vi "Process.vi"(8 "error in (no error)":errorcluster, 10 "DAQ Class.lvclass":refnum<class "DAQ Class.lvclass">, 11 "Intensity Processing in":refnum<class "Intensity Processing.lvclass">) -> (0 "error out":errorcluster, 3 "Intensity Processing out":refnum<class "Intensity Processing.lvclass">)   [LabVIEW 2014, in "Intensity Processing.lvclass"]
uses:
  Intensity Processing.lvclass
  Classes/DAQ/DAQ Class.lvclass
  Classes/DAQ Control Functional Global States.ctl
  <vilib>/Analysis/4window.llb/Hanning Window (DBL).vi
  <vilib>/Analysis/2dsp.llb/Real FFT.vi
  <vilib>/Analysis/4window.llb/AllCosWindow (DBL).vi
  Classes/Processing.lvclass
  <vilib>/Analysis/NI_AALPro.lvlib
panel:
  out "Log?":bool=TRUE
  out "Intensity Graph":dbl[][](graph)
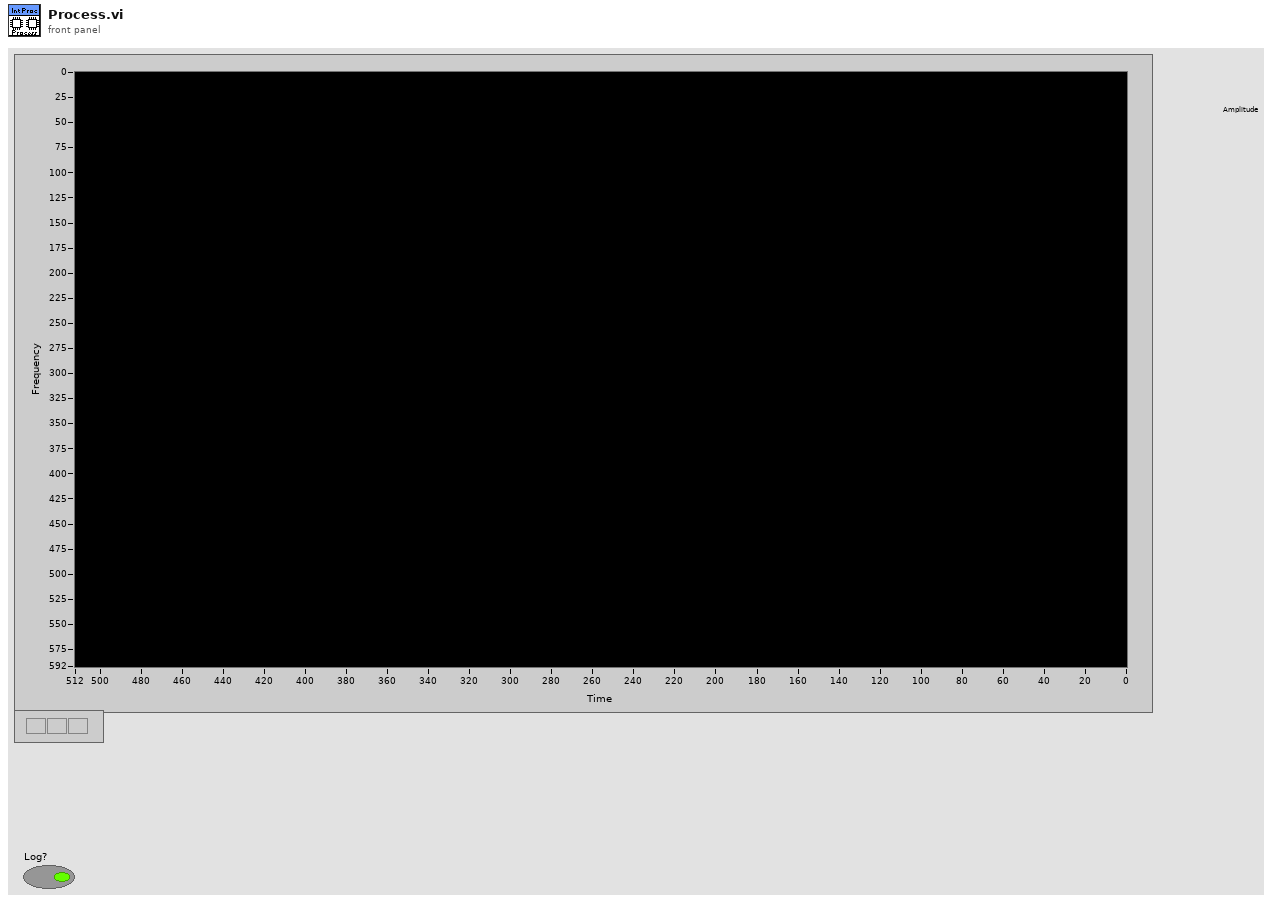
[diagram p1: front panel]
types:
  T1 = typedef "DAQ Class.lvclass/DAQ Parameters.ctl" = cluster{"Points Per A-Scan":u32, "A-Scans Per B-Scan":u32, "Number of B-Scans":u32, "A-Scans Per Transfer":u32, "Trigger Voltage":sgl, "Trigger Source":T2, "Trigger Slope":T3, "Channel":T4, "Clock":T5, "Bits per Sample":dbl, "Range":dbl}
  T2 = typedef "DAQ Class.lvclass/Trigger Source.ctl" = enum16{"External", "Channel A", "Channel B"}
  T3 = typedef "DAQ Class.lvclass/Trigger Slope.ctl" = enum16{"Rising", "Falling"}
  T4 = typedef "OCT DAQ Channel Data Type.ctl" = enum16{"Channel 1", "Channel 2", "Channel 1 and 2"}
  T5 = typedef "DAQ Class.lvclass/Clock Control.ctl" = enum16{"Internal Clock", "External Clock"}
  T6 = enum16{"open", "replace", "create", "open or create", "replace or create", "replace or create with confirmation"}
  T7 = typedef "DAQ Control Functional Global States.ctl" = enum16{"Status", "Set Processing Finished", "Reset", "Clear", "Set DAQ Finished"}
  T8 = typedef "LVCursorListTypeDef.ctl" = cluster{"Name":string, "Color":u32, "Style":u8, "Point Style":u8, "Name Visible":bool, "Allow Drag":bool, "Cursor Mode":u32, "Plot":i32, "Index":i32, "Position":cluster{"X":dbl, "Y":dbl}, "X Scale":u32, "Y Scale":u32, "Watch Plots":i32[], "Watch All Plots":bool, "Plot Area":i32, "Label Offset":cluster{"X":dbl, "Y":dbl}}[]
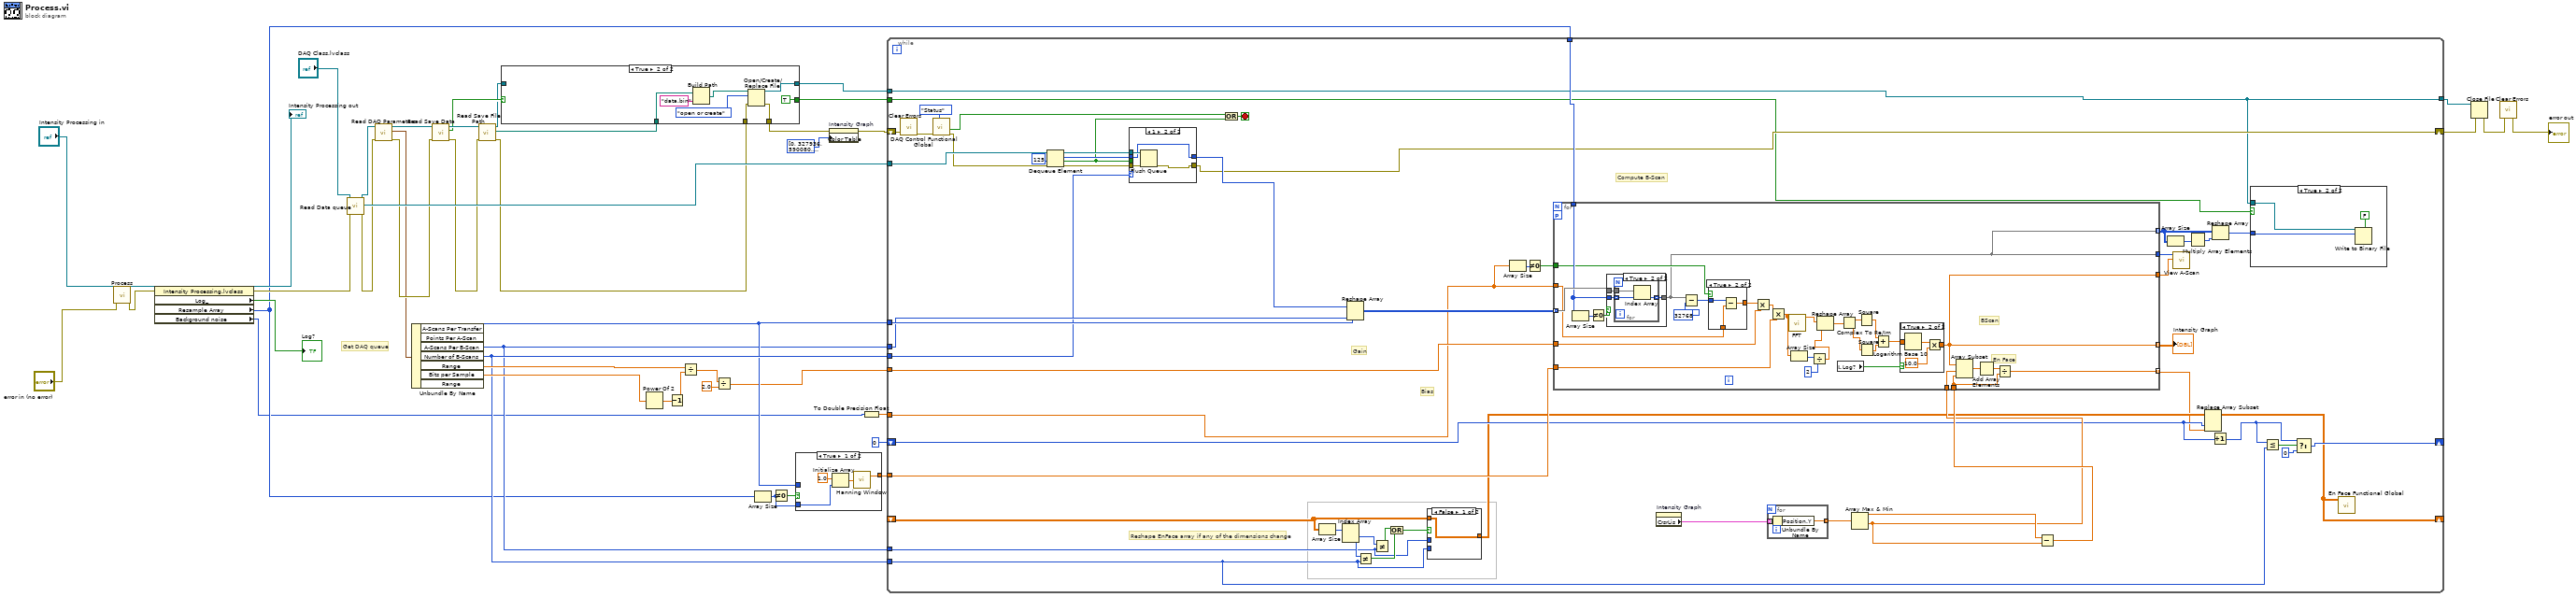
[diagram p0: block diagram]
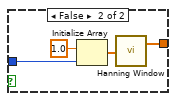
[diagram p2: hidden frame]
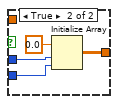
[diagram p9: hidden frame]
diagram:
  # "Get DAQ queue"
  n1 = call-parent "Process.vi"("error in (no error)"="error in (no error)", "Processing in"="Intensity Processing in") -> ("error out"=w24:errorcluster, "Processing out"=w26:refnum<class "Intensity Processing.lvclass">)  [unwired: 8 in]
  n2 = property class="Intensity Processing.lvclass"(reference=w26, error in=w24) -> (reference out=→"Intensity Processing out":refnum<class "Intensity Processing.lvclass">, error out=w23:errorcluster, "Log_"=→"Log?":bool, "Resample Array"=w7:u32[], "Background noise"=w1:u32[])
  n3 = call-dynamic "Read Data queue.vi"("error in (no error)"=w23, "DAQ Class in"="DAQ Class.lvclass") -> ("error out"=w44:errorcluster, "Data queue"=w45:refnum<queue>, "DAQ Class out"=w43:refnum<class "DAQ Class.lvclass">)  [unwired: 7 in]
  n4 = call-dynamic "Read DAQ Parameters.vi"("error in (no error)"=w44, "DAQ Class in"=w43) -> ("error out"=w19:errorcluster, "DAQ Parameters"=w9:T1, "DAQ Class out"=w21:refnum<class "DAQ Class.lvclass">)  [unwired: 7 in]
  n5 = Unbundle By Name(w9) -> ("Points Per A-Scan"=w14:u32, "A-Scans Per B-Scan"=w13:u32, "Number of B-Scans"=w15:u32, "Range"=w40:dbl, "Bits per Sample"=w41:dbl)  [unwired: 2 out]
  n6 = call-dynamic "Read Save Data.vi"("error in (no error)"=w19, "DAQ Class in"=w21) -> ("error out"=w20:errorcluster, "Save Data"=w17:bool, "DAQ Class out"=w18:refnum<class "DAQ Class.lvclass">)  [unwired: 7 in]
  n7 = call-dynamic "Read Save File Path.vi"("error in (no error)"=w20, "DAQ Class in"=w18) -> ("error out"=w33:errorcluster, "Save File Path"=w16:path, "DAQ Class out"=w5:refnum<class "DAQ Class.lvclass">)  [unwired: 7 in]
  n8 = case shown="True" w17 {
    selector: w17 -> [w47 _]
    tunnel: w33 -> [w48 w56]
    tunnel: [w48 w55] -> w11
    tunnel: [_ w54] -> w37
    tunnel: [w47 TRUE] -> w36
    tunnel: w16 -> [_ w52]
    tunnel: w5 -> [_ _]
    frame False {
    }
    frame True {
      n9 = Build Path(base path=w52, name or relative path="data.bin") -> (appended path=w51:path)
      n10 = Open/Create/Replace File(file path (use dialog)=w51, error in=w56, operation (0:open)=T6."open or create") -> (refnum out=w54:refnum<file>, error out=w55:errorcluster)  [unwired: 3 in, 1 out]
    }
  }
  n11 = Power Of 2(x=w41) -> (2^x=w42:dbl)
  n12 = Decrement(x=w42) -> (x-1=w39:dbl)
  n13 = Divide(x=w40, y=w39) -> (x/y=w4:dbl)
  n14 = Divide(x=w4, y=2.0) -> (x/y=w3:dbl)
  n15 = Array Size(array=w7) -> (size(s)=w6:i32)
  n16 = Not Equal To 0?(x=w6) -> (x != 0?=w8:bool)
  n17 = case shown="True" w8 {
    tunnel: [w58 w62] -> w31
    tunnel: w14 -> [_ w61]
    tunnel: w6 -> [w57 _]
    frame True {
      n18 = Initialize Array(1.0 ("element"), w57) -> (w60:dbl[])
      n19 = call-poly <vilib>:"Hanning Window.vi"("X"=w60) -> ("Windowed X"=w58:dbl[])  [unwired: 1 out]
    }
    frame False {
      n20 = Initialize Array(1.0 ("element"), w61) -> (w64:dbl[])
      n21 = call-poly <vilib>:"Hanning Window.vi"("X"=w64) -> ("Windowed X"=w62:dbl[])  [unwired: 1 out]
    }
  }
  n22 = property on="Intensity Graph" class="IntGraph (strict)"(error in=w11, "Color Table"=u32[] [0, 327936, 590080, 852224, 983296, 1114624, 1180160, 1311232, 1442304, 1573632, 1704704, 1770240, 1901312, 1966848, 2098176, 2163712, 2294784, 2491392, 2557184, 2688256, 2753792, 2884864, 2950656, 3081728, 3147264, 3344129, 3475457, 3540993, 3672321, 3738113, 3869185, 3934977, 4066305, 4197633, 4328961, 4394497, 4460289, 4591617, 4657409, 4788481, 4854273, 4985601, 5116929, 5248257, 5314049, 5379841, 5511169, 5576961, 5708033, 5773825, 5905153, 6036482, 6167810, 6233346, 6299138, 6430466, 6496258, 6562050, 6693634, 6759426, 6890754, 7022082, 7087874, 7153666, 7284994, 7350786, 7482114, 7547906, 7613698, 7745026, 7876354, 8007682, 8073474, 8139522, 8205314, 8336642, 8467970, 8533763, 8599555, 8665347, 8731139, 8862467, 8993795, 9059587, 9125380, 9191428, 9257220, 9388548, 9454340, 9520132, 9585924, 9717253, 9848837, 9914629, 9980165, 10045957, 10177541, 10243334, 10309126, 10375174, 10440966, 10572294, 10703623, 10769416, 10835208, 10901256, 10967049, 11033097, 11033609, 11099401, 11165450, 11231242, 11231754, 11297547, 11363339, 11429131, 11495180, 11495692, 11561740, 11693069, 11758861, 11759373, 11825165, 11891214, 11957006, 12022799, 12023311, 12089103, 12220944, 12286736, 12286736, 12352529, 12418577, 12484370, 12550162, 12615954, 12681747, 12747796, 12813588, 12813845, 12879894, 12945686, 13077015, 13142808, 13143064, 13208856, 13274905, 13340697, 13340953, 13472282, 13538075, 13604379, 13670172, 13735964, 13801757, 13867550, 13933343, 13999392, 13999648, 14065441, 14131234, 14197027, 14197541, 14263334, 14329383, 14395176, 14460969, 14592553, 14658346, 14724139, 14789932, 14790189, 14856238, 14922287, 14988080, 15053873, 15054130, 15119923, 15185972, 15251765, 15317559, 15383353, 15449146, 15449660, 15515454, 15515968, 15516226, 15582021, 15582278, 15582536, 15648587, 15648844, 15714639, 15714897, 15715155, 15780949, 15781463, 15847256, 15847770, 15848028, 15913823, 15914081, 15979875, 15980133, 15980391, 16046441, 16046444, 16046703, 16046705, 16112500, 16113015, 16113274, 16113277, 16179072, 16179330, 16179588, 16245384, 16245387, 16245389, 16245648, 16311443, 16376982, 16377241, 16377499, 16443294, 16443553, 16443555, 16443815, 16509866, 16510124, 16510127, 16575923, 16575924, 16576182, 16576441, 16576443, 16576702, 16576705, 16576963, 16577222, 16577224, 16577482, 16577485, 16577743, 16577745, 16578004, 16578262, 16578264, 16578523, 16578782, 16579040, 16579299, 16579301, 16579303, 16579562, 16579821]) -> (error out=w12:errorcluster)  [unwired: 1 in, 1 out]
  n23 = To Double Precision Float(number=w1) -> (double precision float=w2:dbl[])
  n24 = while {
    tunnel: w45 -> [w91]
    shift-right: [w82] -> w35
    shift-left: w12 -> [w118]
    tunnel: w3 -> [w87]
    tunnel: w14 -> [w97]
    tunnel: w13 -> [w96]
    tunnel: w31 -> [w119]
    tunnel: w37 -> [w68]
    tunnel: w36 -> [w67]
    tunnel: [w68] -> w34
    shift-right: [w106] -> _
    shift-left: _ -> [w105]
    shift-right: [w110] -> _
    shift-left: 0 -> [w111]
    tunnel: w13 -> [w98]
    tunnel: w15 -> [w86]
    tunnel: w15 -> [w66]
    tunnel: w7 -> [w85]
    tunnel: w2 -> [w73]
    stop <- w109 stop-if-true
    # "Compute B-Scan"
    # "Reshape EnFace array if any of the dimensions change"
    # "Bias"
    # "Gain"
    n25 = call <vilib>:"Clear Errors.vi"("error in (no error)"=w118) -> ("error out"=w117:errorcluster)  [unwired: 5 in, 1 out]
    n26 = call "DAQ Control Functional Global.vi"("State"=DAQ_Control_Functional_Global_States."Status", "Error In"=w117) -> ("Error Out"=w90:errorcluster, "Reset?"=w92:bool)  [unwired: 6 in, 2 out]
    n27 = Dequeue Element(queue=w91, timeout in ms (-1)=125, error in (no error)=w90) -> (queue out=w76:refnum<queue>, element=w77:u16[], timed out?=w65:bool, error out=w75:errorcluster)
    n28 = case shown="1" w66 {
      tunnel: w77 -> [w124 w125]
      tunnel: w76 -> [_ w127]
      tunnel: [w124 w125] -> w89
      tunnel: w65 -> [_ _]
      tunnel: w75 -> [w123 w128]
      tunnel: [w123 w126] -> w82
      frame 0, Default {
      }
      frame 1 {
        n29 = Flush Queue(queue=w127, error in (no error)=w128) -> (error out=w126:errorcluster)  [unwired: 2 out]
      }
    }
    n30 = Or(x=w92, y=w65) -> (x .or. y?=w109:bool)
    n31 = Array Size(array=w105) -> (size(s)=w104:i32[])
    n32 = Index Array(array=w104) -> (element #1=w102:i32, element #2=w103:i32)  [unwired: 2 in]
    n33 = Reshape Array(w89, w96, w97) -> (w88:u16[][])
    n34 = Not Equal?(x=w103, y=w86) -> (x != y?=w100:bool)
    n35 = Not Equal?(x=w102, y=w98) -> (x != y?=w99:bool)
    n36 = Or(x=w99, y=w100) -> (x .or. y?=w101:bool)
    n37 = case shown="False" w101 {
      tunnel: w98 -> [_ w179]
      tunnel: w86 -> [_ w178]
      tunnel: [w176 w177] -> w107
      tunnel: w105 -> [w176 _]
      frame False {
      }
      frame True {
        n38 = Initialize Array(0.0 ("element"), w179, w178) -> (w177:dbl[][])
      }
    }
    n39 = Array Size(array=w73) -> (size(s)=w84:i32)
    n40 = Not Equal To 0?(x=w84) -> (x != 0?=w83:bool)
    n41 = property on="Intensity Graph" class="IntGraph (strict)"() -> ("CrsrLis"=w113:T8)  [unwired: 2 in, 2 out]
    n42 = for {
      tunnel: w113 -> [w182] mode=indexing
      tunnel: [w181] -> w112 mode=indexing
      n43 = Unbundle By Name(w182) -> ("Position.Y"=w181:dbl)
    }
    n44 = Array Max & Min(array=w112) -> (max value=w116:dbl, min value=w114:dbl)  [unwired: 2 out]
    n45 = Subtract(x=w116, y=w114) -> (x-y=w115:dbl)
    n46 = for {
      tunnel: w119 -> [w159]
      tunnel: [w130] -> w74 mode=indexing
      tunnel: w115 -> [w148]
      tunnel: w114 -> [w151]
      tunnel: [w147] -> w81 mode=indexing
      tunnel: w87 -> [w145]
      tunnel: w88 -> [w144] mode=indexing
      tunnel: w85 -> [w140]
      tunnel: w73 -> [w133]
      tunnel: w83 -> [w131]
      tunnel: [w130] -> w80
      tunnel: [w129] -> w79
      tunnel: [w129] -> w72 mode=indexing
      workers-P: _ -> [_]
      # "BScan"
      # "En Face"
      n47 = Array Size(array=w140) -> (size(s)=w139:i32)
      n48 = Not Equal To 0?(x=w139) -> (x != 0?=w138:bool)
      n49 = case shown="True" w138 {
        tunnel: w140 -> [_ w167]
        tunnel: w144 -> [w164 w166]
        tunnel: [w164 w165] -> w129
        frame False {
        }
        frame True {
          n50 = for {
            tunnel: w167 -> [w169] mode=indexing
            tunnel: w166 -> [w170]
            tunnel: [w168] -> w165 mode=indexing
            n51 = Index Array(array=w170, index=w169) -> (element=w168:u16)
          }
        }
      }
      n52 = Subtract(x=w129, y=32768) -> (x-y=w134:i32[])
      n53 = case shown="True" w131 {
        tunnel: w134 -> [w160 w163]
        tunnel: w133 -> [_ w162]
        tunnel: [w160 w161] -> w132
        frame False {
        }
        frame True {
          n54 = Subtract(x=w163, y=w162) -> (x-y=w161:dbl[])
        }
      }
      n55 = Multiply(x=w132, y=w145) -> (x*y=w135:dbl[])
      n56 = Multiply(x=w135, y=w159) -> (x*y=w137:dbl[])
      n57 = call-poly <vilib>:"FFT.vi"("X"=w137) -> ("FFT {X}"=w153:cdb[])  [unwired: 9 in, 1 out]
      n58 = Array Size(array=w137) -> (size(s)=w143:i32)
      n59 = Divide(x=w143, y=2) -> (x/y=w141:dbl)
      n60 = Reshape Array(w153, w141) -> (w152:cdb[])
      n61 = local read "Log?"() -> (w146:bool)
      n62 = Complex To Re/Im(x + iy=w152) -> (x=w158:dbl[], y=w157:dbl[])
      n63 = Square(x=w158) -> (x^2=w156:dbl[])
      n64 = Square(x=w157) -> (x^2=w155:dbl[])
      n65 = Add(x=w156, y=w155) -> (x+y=w154:dbl[])
      n66 = case shown="True" w146 {
        tunnel: w154 -> [w171 w175]
        tunnel: [w171 w172] -> w130
        frame False {
        }
        frame True {
          n67 = Logarithm Base 10(1:w175) -> (0:w174:dbl[])
          n68 = Multiply(x=w174, y=10.0 ("element")) -> (x*y=w172:dbl[])
        }
      }
      n69 = Array Subset(array=w130, index=w151, length=w148) -> (w150:dbl[])
      n70 = Add Array Elements(numeric array=w150) -> (sum=w149:dbl)
      n71 = Divide(x=w149, y=w148) -> (x/y=w147:dbl)
    }
    "Intensity Graph" <- w74
    n72 = Array Size(array=w72) -> (size(s)=w70:i32[])
    n73 = call "View A-Scan.vi"("A-Scan Processed"=w80, "A-Scan (Raw)"=w79) -> ()  [unwired: 10 in]
    n74 = Multiply Array Elements(1:w70) -> (0:w71:i32)
    n75 = Replace Array Subset(array=w107, new element=w81, index (col)=w111) -> (w106:dbl[][])  [unwired: 1 in]
    n76 = Increment(x=w111) -> (x+1=w94:i32)
    n77 = Reshape Array(w72, w71) -> (w69:u16[])
    n78 = case shown="True" w67 {
      tunnel: w68 -> [_ w121]
      tunnel: w69 -> [_ w120]
      frame False {
      }
      frame True {
        n79 = Write to Binary File(file (use dialog)=w121, data=w120, 5:FALSE ("prepend array or string size? (T)")) -> ()  [unwired: 3 in, 3 out]
      }
    }
    n80 = Less Or Equal?(x=w94, y=w86) -> (x <= y?=w95:bool)
    n81 = Select(t=w94, s=w95, f=0) -> (s? t:f=w110:i32)
    n82 = call "En Face Functional Global.vi"("Intensity Graph 2"=w106) -> ()  [unwired: 9 in, 2 out]
  }
  n83 = Close File(refnum=w34, error in=w35) -> (error out=w29:errorcluster)  [unwired: 1 out]
  n84 = call <vilib>:"Clear Errors.vi"("error in (no error)"=w29) -> ("error out"=→"error out":errorcluster)  [unwired: 5 in, 1 out]
